vi "Write String.vi"(8 "error in (no error)":errorcluster, 10 "String":string, 11 "NI DA in":refnum<class "NI Digital to Analog.lvclass">) -> (0 "error out":errorcluster, 3 "NI DA out":refnum<class "NI Digital to Analog.lvclass">)   [LabVIEW 2018, in "NI Digital to Analog.lvclass"]
doc: "Bus.lvclass:Read String.vi\n\nThis is the template for the Read String VI forthe Bus class.\n\nInstrument Communication Module Version 1.0\nJuly, 2017 Original Code Consulting David Thomson\n www.originalcode.com"
uses:
  NI Digital to Analog.lvclass
  NI Digital to Analog.lvclass/NI Digital to Analog.ctl
  <vilib>/DAQmx/write.llb/DAQmx Write (Analog 1D DBL NChan 1Samp).vi
  <vilib>/DAQmx/miscellaneous.llb/DAQmx Fill In Error Info.vi
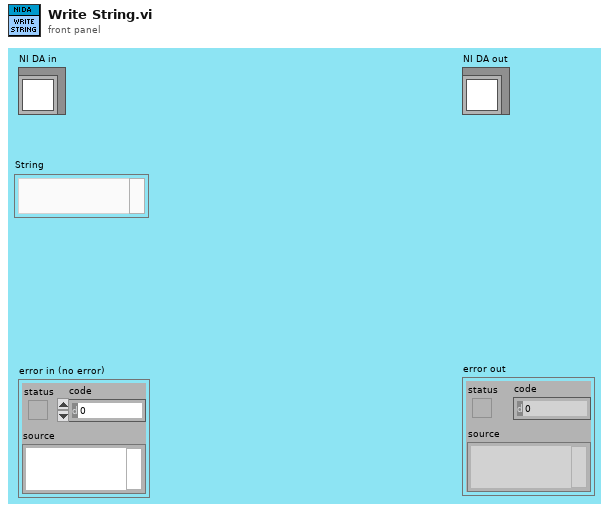
[diagram p1: front panel]
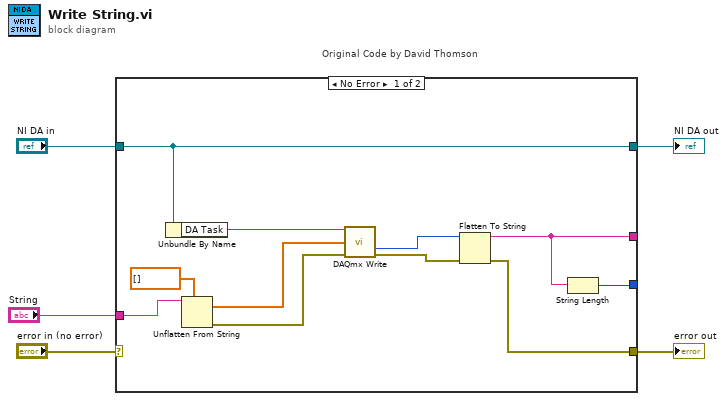
[diagram p0: block diagram]
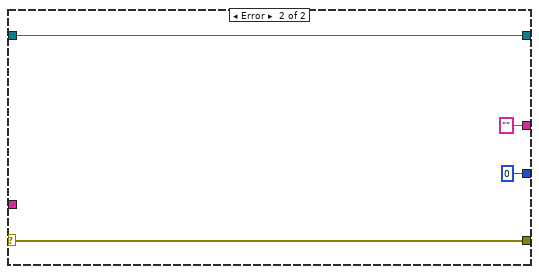
[diagram p2: hidden frame]
diagram:
  n1 = case "Original Code by David Thomson" shown="No Error" "error in (no error)" {
    selector: "error in (no error)" -> [_ w20]
    tunnel: [w12 w20] -> w4
    tunnel: [w15 w19] -> w3
    tunnel: "NI DA in" -> [w15 w19]
    tunnel: [w11 ""] -> _
    tunnel: [w10 0] -> _
    tunnel: "String" -> [w9 _]
    frame No Error {
      n2 = Unbundle By Name(w15) -> ("DA Task"=w16:refnum<k21>)
      n3 = Unflatten From String(type=dbl[] [] ("array type (2D Dbl)"), binary string=w9) -> (value=w8:dbl[], error out=w6:errorcluster)  [unwired: 3 in, 1 out]
      n4 = call-poly <vilib>:"DAQmx Write.vi"("task/channels in"=w16, "data"=w8, "error in"=w6) -> ("number of samples written per channel"=w14:u32, "error out"=w13:errorcluster)  [unwired: 10 in, 1 out]
      n5 = Flatten To String(anything=w14, error in (no error)=w13) -> (data string=w11:string, error out=w12:errorcluster)  [unwired: 2 in, 1 out]
      n6 = String Length(string=w11) -> (length=w10:i32)
    }
    frame Error {
    }
  }
  "error out" <- w4
  "NI DA out" <- w3
